vi "Adaptive Thresholding.vi"(8 "error in":errorcluster, 9 "Steps":i32=36, 10 "PFA":dbl, 11 "Spectrum Data":cluster{"Mags":dbl[], "Freq":dbl[]}) -> (0 "error out":errorcluster, 2 "Noise Floor":dbl[](array[numeric]), 3 "Threshold Data":cluster{"Mags":dbl[], "Freq":dbl[]})   [LabVIEW 2019]
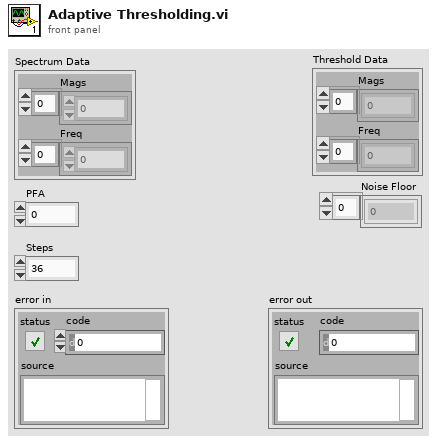
[diagram p1: front panel]
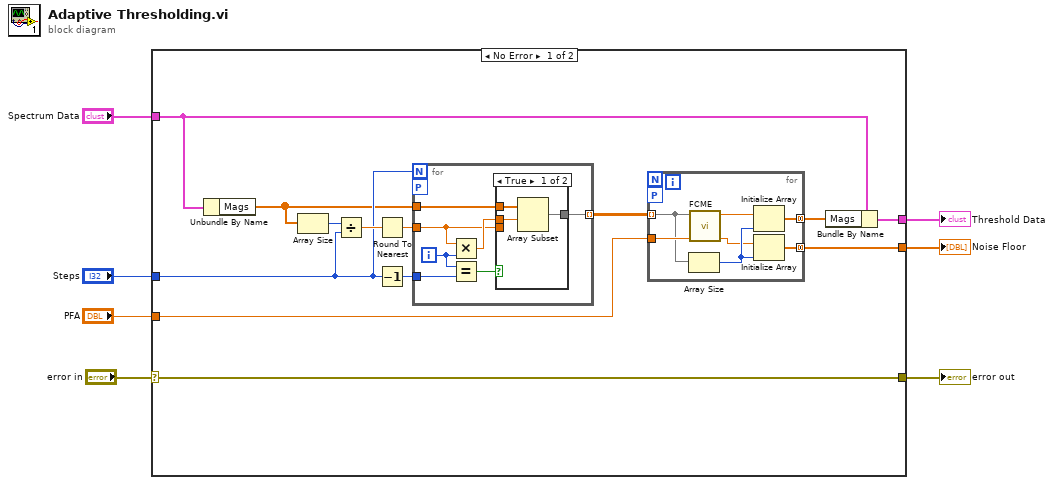
[diagram p0: block diagram]
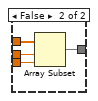
[diagram p2: hidden frame]
diagram:
  n1 = case shown="No Error" "error in" {
    selector: "error in" -> [w8 w42]
    tunnel: "Steps" -> [w18 _]
    tunnel: "PFA" -> [w13 _]
    tunnel: [w11 _] -> w5
    tunnel: "Spectrum Data" -> [w10 _]
    tunnel: [w9 _] -> w3
    tunnel: [w8 w42] -> w1
    frame No Error {
      n2 = Unbundle By Name(w10) -> ("Mags"=w12:dbl[])
      n3 = Array Size(array=w12) -> (size(s)=w20:i32)
      n4 = Divide(x=w20, y=w18) -> (x/y=w19:dbl)
      n5 = Round To Nearest(number=w19) -> (nearest integer value=w16:dbl)
      n6 = Decrement(x=w18) -> (x-1=w17:i32)
      n7 = for {
        N: w18 -> [_]
        tunnel: w12 -> [w34]
        tunnel: w16 -> [w32]
        tunnel: [w31] -> w14 mode=indexing
        tunnel: w17 -> [w28]
        workers-P: _ -> [_]
        i -> [w29]
        n8 = Multiply(x=w32, y=w29) -> (x*y=w33:dbl)
        n9 = Equal?(x=w29, y=w28) -> (x = y?=w30:bool)
        n10 = case shown="True" w30 {
          tunnel: w34 -> [w37 w41]
          tunnel: w33 -> [w36 w39]
          tunnel: w32 -> [_ w38]
          tunnel: [w35 w40] -> w31
          frame True {
            n11 = Array Subset(array=w37, index=w36) -> (w35:dbl[])  [unwired: 1 in]
          }
          frame False {
            n12 = Array Subset(array=w41, index=w39, length=w38) -> (w40:dbl[])
          }
        }
      }
      n13 = for {
        tunnel: w14 -> [w26] mode=indexing
        workers-P: _ -> [_]
        tunnel: w13 -> [w27]
        tunnel: [w25] -> w15 mode=concatenating
        tunnel: [w22] -> w9 mode=concatenating
        n14 = Array Size(array=w26) -> (size(s)=w23:i32)
        n15 = call "FCME.vi"("PFA"=w27, "Mag"=w26) -> ("Noise Floor"=w21:dbl, "Threshold"=w24:dbl)  [unwired: 8 in]
        n16 = Initialize Array(w24, w23) -> (w25:dbl[])
        n17 = Initialize Array(w21, w23) -> (w22:dbl[])
      }
      n18 = Bundle By Name(cluster=w10, "Mags"=w15) -> (w11:cluster{"Mags":dbl[], "Freq":dbl[]})
    }
    frame Error {
    }
  }
  "Threshold Data" <- w5
  "Noise Floor" <- w3
  "error out" <- w1
